vi "Config-Receiver.vi"(8 "error in":errorcluster, 11 "Refnum in":T1) -> (0 "error out":errorcluster, 2 "Receiver":T2, 3 "Refnum out":T1)   [LabVIEW 2021, in "UDP_Config.lvclass"]
uses:
  UDP_Config.lvclass
  Receiver.ctl
  <vilib>/Utility/config.llb/Config Data RefNum.ctl
  <vilib>/Utility/config.llb/Read Key (I32).vi
  <vilib>/Utility/config.llb/Read Key (String).vi
  <vilib>/Utility/config.llb/Read Key (U32).vi
  <vilib>/Utility/config.llb/NI_LVConfig.lvlib
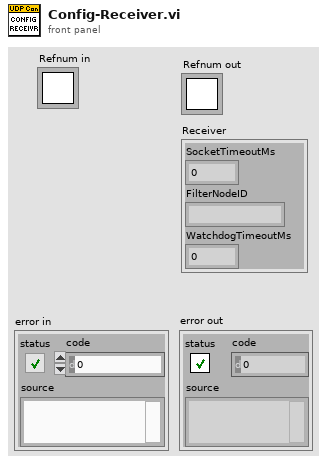
[diagram p1: front panel]
types:
  T1 = typedef "NI_LVConfig.lvlib/Config Data RefNum.ctl" = refnum<k1>
  T2 = typedef "Receiver.ctl" = cluster{"SocketTimeoutMs":i32, "FilterNodeID":string, "WatchdogTimeoutMs":u32}
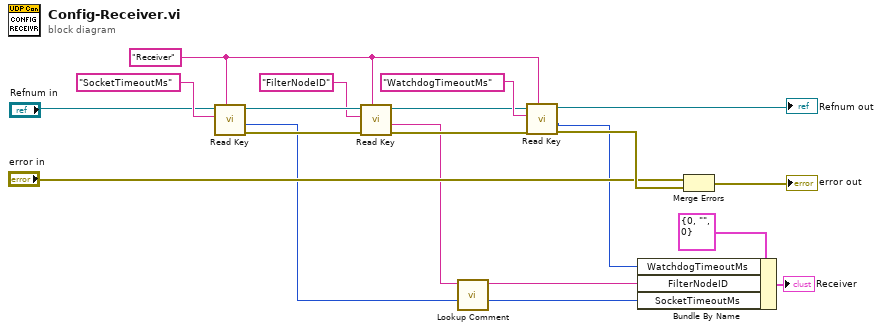
[diagram p0: block diagram]
diagram:
  w17 = "Receiver" ("key")
  n1 = call-poly <vilib>:"Read Key.vi"("section"=w17, "key"="SocketTimeoutMs", "refnum"="Refnum in") -> ("error out"=w10:errorcluster, "value"=w3:i32, "refnum out"=w12:T1)  [unwired: 5 in, 1 out]
  n2 = call-poly <vilib>:"Read Key.vi"("section"=w17, "error in (no error)"=w10, "key"="FilterNodeID", "refnum"=w12) -> ("error out"=w16:errorcluster, "value"=w5:string, "refnum out"=w15:T1)  [unwired: 4 in, 1 out]
  n3 = call "Lookup Comment.vi"("String in"=w5) -> ("Value"=w4:string)  [unwired: 3 in, 1 out]
  n4 = call-poly <vilib>:"Read Key.vi"("section"=w17, "error in (no error)"=w16, "key"="WatchdogTimeoutMs", "refnum"=w15) -> ("error out"=w9:errorcluster, "value"=w1:u32, "refnum out"=→"Refnum out":T1)  [unwired: 4 in, 1 out]
  n5 = Bundle By Name(cluster=T2 {"SocketTimeoutMs"=0, "FilterNodeID"="", "WatchdogTimeoutMs"=0} ("Receiver"), "WatchdogTimeoutMs"=w1, "FilterNodeID"=w4, "SocketTimeoutMs"=w3) -> (→"Receiver":T2)
  n6 = Merge Errors("error in", w9) -> (→"error out":errorcluster)
